vi "Create Resources.vi"() -> (4 "address space collection":refnum<class "Address Space Collection.lvclass">, 15 "stream control session":refnum<class "niUSRP Sync v1 FPGA.lvclass">)   [LabVIEW 2025, in "niUSRP Sync v1 FPGA.lvclass"]
uses:
  niUSRP Sync v1 FPGA.lvclass
  C:/Program Files/NI/LVAddons/niidl/1/instr.lib/_niInstr/Instruction Framework/v1/FPGA/Interfaces/Address Space/Address Space.lvclass
  <instrlib>/_niInstr/Instruction Framework/v1/FPGA/Interfaces/Address Space Collection/Address Space Collection.lvclass
  niUSRP Sync v1 FPGA.lvclass/niUSRP Sync v1 FPGA.ctl
  <instrlib>/_niInstr/Instruction Framework/v1/FPGA/Helper Classes/Single Address Space Collection/Single Address Space Collection.lvclass
  C:/Program Files/NI/LVAddons/niidl/1/instr.lib/_niInstr/Instruction Framework/v1/FPGA/Interfaces/Address Space Collection/Address Space Collection.lvclass
  <vilib>/rvi/DataTransferAndStorage/Container/Common/niFpgaContainerGetUniqueNameForEmu.vi
  <vilib>/rvi/DataTransferAndStorage/Container/Common/niFpgaContainerSetEmuInfo.vi
  <vilib>/rvi/eio/common/nirviEmuReportErrorAndStop.vi
  <vilib>/rvi/LocalResourceManager/LocalResourceManager.xnode
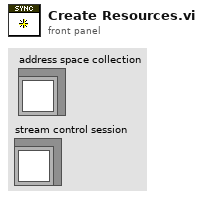
[diagram p1: front panel]
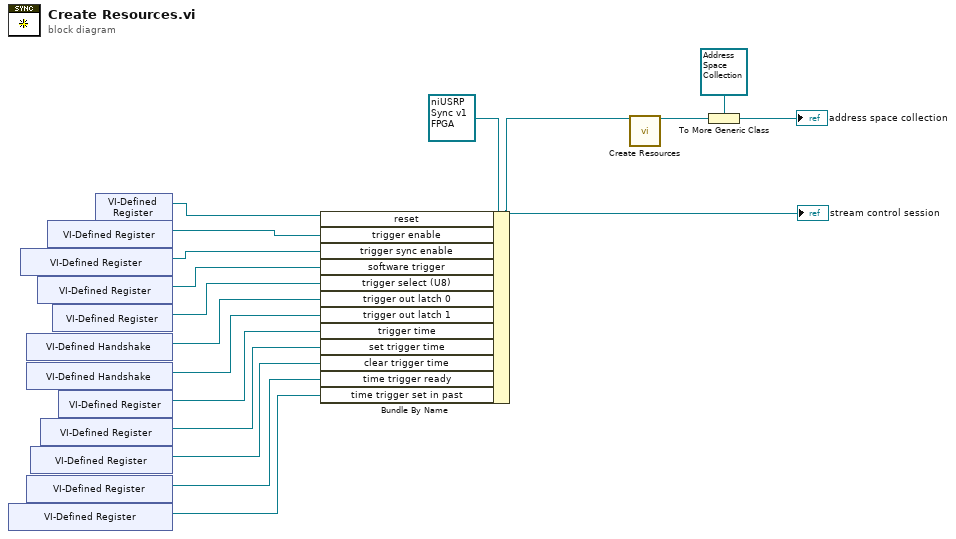
[diagram p0: block diagram]
diagram:
  n1 = xnode "VI-Defined Register"() -> ("Register Out"=w1:refnum<k21>)
  n2 = xnode "VI-Defined Register"() -> ("Register Out"=w11:refnum<k21>)
  n3 = xnode "VI-Defined Handshake"() -> ("Handshake Out"=w7:refnum<k21>)
  n4 = xnode "VI-Defined Handshake"() -> ("Handshake Out"=w6:refnum<k21>)
  n5 = xnode "VI-Defined Register"() -> ("Register Out"=w2:refnum<k21>)
  n6 = xnode "VI-Defined Register"() -> ("Register Out"=w3:refnum<k21>)
  n7 = xnode "VI-Defined Register"() -> ("Register Out"=w10:refnum<k21>)
  n8 = xnode "VI-Defined Register"() -> ("Register Out"=w4:refnum<k21>)
  n9 = xnode "VI-Defined Register"() -> ("Register Out"=w12:refnum<k21>)
  n10 = xnode "VI-Defined Register"() -> ("Register Out"=w9:refnum<k21>)
  n11 = xnode "VI-Defined Register"() -> ("Register Out"=w5:refnum<k21>)
  n12 = xnode "VI-Defined Register"() -> ("Register Out"=w8:refnum<k21>)
  n13 = Bundle By Name(cluster=refnum<class "niUSRP Sync v1 FPGA.lvclass"> refnum ("niUSRP Stream Control v1 FPGA.lvclass"), "reset"=w8, "trigger enable"=w12, "trigger sync enable"=w11, "software trigger"=w10, "trigger select (U8)"=w9, "trigger out latch 0"=w7, "trigger out latch 1"=w6, "trigger time"=w5, "set trigger time"=w4, "clear trigger time"=w3, "time trigger ready"=w2, "time trigger set in past"=w1) -> (w14:refnum<class "niUSRP Sync v1 FPGA.lvclass">)
  "stream control session" <- w14
  n14 = call <instrlib>:"Create Resources.vi"("address space"=w14) -> ("single address space collection"=w13:refnum<class "Single Address Space Collection.lvclass">)  [unwired: 14 in]
  n15 = To More Generic Class(target class=refnum<class "Address Space Collection.lvclass"> refnum ("collection"), reference=w13) -> (generic class reference=→"address space collection":refnum<class "Address Space Collection.lvclass">)
